vi "创建脚本文件.vi"(8 "错误输入":errorcluster) -> (0 "错误输出":errorcluster)   [LabVIEW 2016, in "数据传输系统-03.lvlib"]
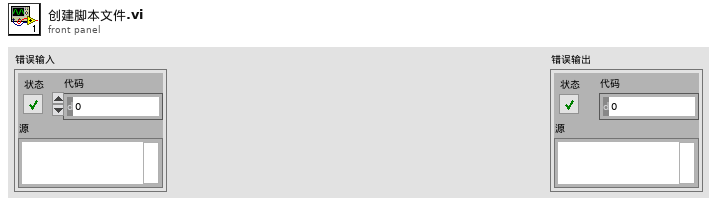
[diagram p1: front panel]
types:
  T1 = enum16{"open", "replace", "create", "open or create", "replace or create", "replace or create with confirmation"}
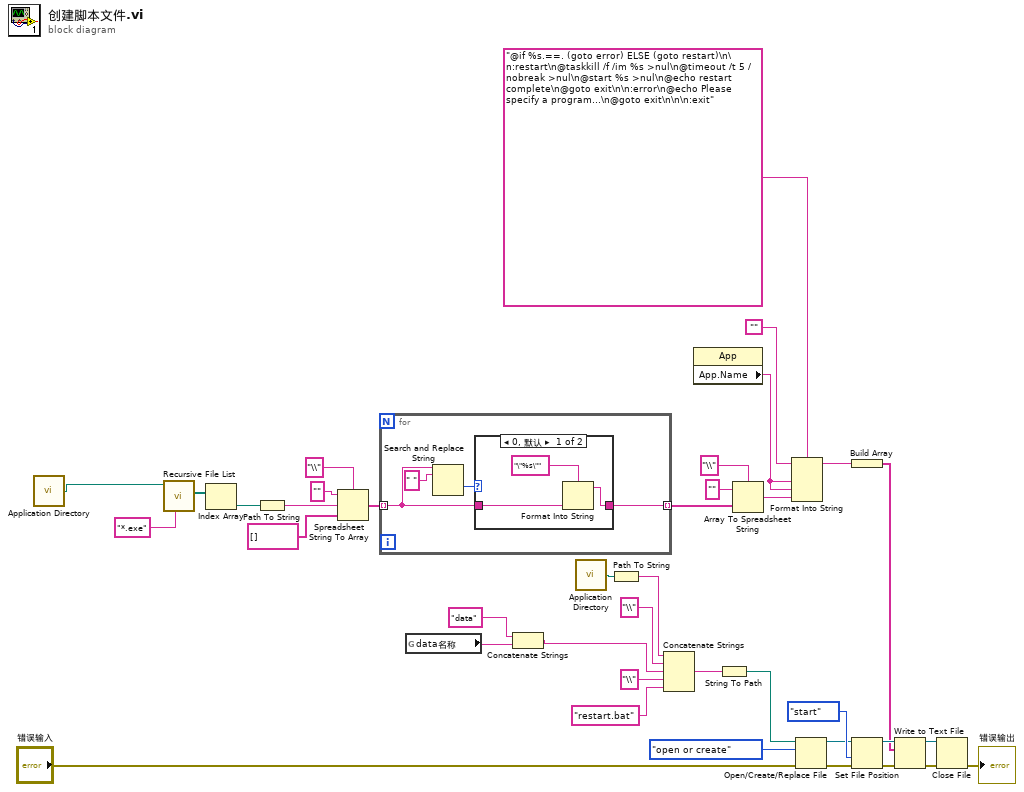
[diagram p0: block diagram]
diagram:
  n1 = call <vilib>:"Application Directory.vi"() -> ("Application Directory"=w14:path)
  n2 = call <vilib>:"Recursive File List.vi"("pattern"="*.exe", "Folder Path"=w14) -> ("All Files in Dir"=w16:path[])  [unwired: 5 in, 4 out]
  n3 = Index Array(array=w16) -> (element=w13:path)  [unwired: 1 in]
  n4 = Path To String(path=w13) -> (string=w5:string)
  n5 = Spreadsheet String To Array(delimiter (Tab)="\\" ("分隔符(Tab)"), format string="" ("格式字符串"), spreadsheet string=w5, array type (2D Dbl)=string[] []) -> (array=w9:string[])
  n6 = for {
    tunnel: w9 -> [w40] mode=indexing
    tunnel: [w39] -> w8 mode=indexing
    n7 = Search and Replace String(input string=w40, search string=" " ("搜索字符串")) -> (offset past replacement=w41:i32)  [unwired: 6 in, 3 out]
    n8 = case shown="0, 默认" w41 {
      tunnel: w40 -> [w44 w46]
      tunnel: [w43 w46] -> w39
      frame 0, Default {
        n9 = Format Into String(format string="\"%s\"" ("格式字符串"), w44) -> (resulting string=w43:string)  [unwired: 2 in, 1 out]
      }
      frame -1 {
      }
    }
  }
  n10 = global read "断电保存全局.vi" "data名称"() -> (w2:string)
  n11 = Concatenate Strings("data" ("名称或相对路径"), w2) -> (w1:string)
  n12 = call <vilib>:"Application Directory.vi"() -> ("Application Directory"=w30:path)
  n13 = Path To String(path=w30) -> (string=w28:string)
  n14 = Concatenate Strings(w28, "\\" ("字符串"), w1, "\\" ("字符串"), "restart.bat" ("字符串")) -> (w25:string)
  n15 = property class="App"() -> ("App.Name"=w19:string)  [unwired: 2 in, 2 out]
  n16 = String To Path(string=w25) -> (path=w21:path)
  n17 = Array To Spreadsheet String(delimiter (Tab)="\\" ("分隔符(Tab)"), array=w8, 3:"" ("格式字符串")) -> (spreadsheet string=w4:string)
  n18 = Format Into String(format string="@if %s.==. (goto error) ELSE (goto restart)\n\n:restart\n@taskkill /f /im %s >nul\n@timeout /t 5 /nobreak >nul\n@start %s >nul\n@echo restart complete\n@goto exit\n\n:error\n@echo Please specify a program...\n@goto exit\n\n\n:exit", initial string="", w19, w19, w4) -> (resulting string=w23:string)  [unwired: 1 in, 1 out]
  n19 = Open/Create/Replace File(file path (use dialog)=w21, error in="错误输入", operation (0:open)=T1."open or create" ("操作(0:open)")) -> (refnum out=w34:refnum<file>, error out=w35:errorcluster)  [unwired: 3 in, 1 out]
  n20 = Build Array(w23) -> (w22:string[])
  n21 = Set File Position(refnum=w34, from (0:start)=enum16{"start", "end", "current"}."start" ("自（0:起始）"), error in=w35) -> (refnum out=w36:refnum<file>, error out=w37:errorcluster)  [unwired: 1 in]
  n22 = Write to Text File(file (use dialog)=w36, text=w22, error in=w37) -> (refnum out=w32:refnum<file>, error out=w31:errorcluster)  [unwired: 1 in, 1 out]
  n23 = Close File(refnum=w32, error in=w31) -> (error out=→"错误输出":errorcluster)  [unwired: 1 out]
